vi "XL320_Read Address.vi"(0 "VISA resource name":refnum<visa-resource-name>, 5 "Motor ID (0)":u8, 7 "Address number (0)":u16 max=49, 9 "Number of Addresses to read (1)":u16=1, 11 "Error in (no error)":errorcluster) -> (4 "VISA resource name Out":refnum<visa-resource-name>, 6 "Data Read":u8[](array[numeric]), 10 "Motor Error Status":T1, 15 "error out":errorcluster)   [LabVIEW 2017, in "Dynamixel XL320.lvlib"]
doc: "Reads an arbitrary number of consecutive addresses from a motor's register. This is a Low-Level VI that is used by other VIs."
uses:
  <instrlib>/Dynamixel XL320 (Drivers instrument)/Dynamixel XL320.lvlib
  <instrlib>/Dynamixel XL320 (Drivers instrument)/Public/Motor Operation/Low Level/XL320_Alarm Setting.ctl
  <instrlib>/Dynamixel XL320 (Drivers instrument)/Public/Configure/XL320_Select_Action.ctl
panel:
  # "Ghislain REMY, IUT de Cachan, 2015 December 2015"
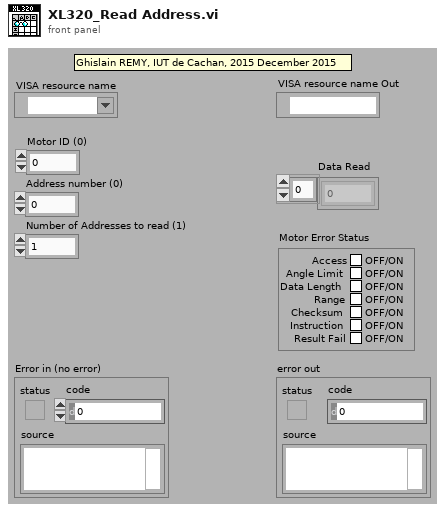
[diagram p1: front panel]
types:
  T1 = typedef "Dynamixel XL320.lvlib/XL320_Alarm Setting.ctl" = cluster{"Access":bool, "Angle Limit":bool, "Data Length":bool, "Range":bool, "Checksum":bool, "Instruction":bool, "Result Fail":bool}
  T2 = cluster{"Boolean array[0]":bool, "Boolean array[1]":bool, "Boolean array[2]":bool, "Boolean array[3]":bool, "Boolean array[4]":bool, "Boolean array[5]":bool, "Boolean array[6]":bool}
  T3 = typedef "Dynamixel XL320.lvlib/XL320_Select_Action.ctl" = u8
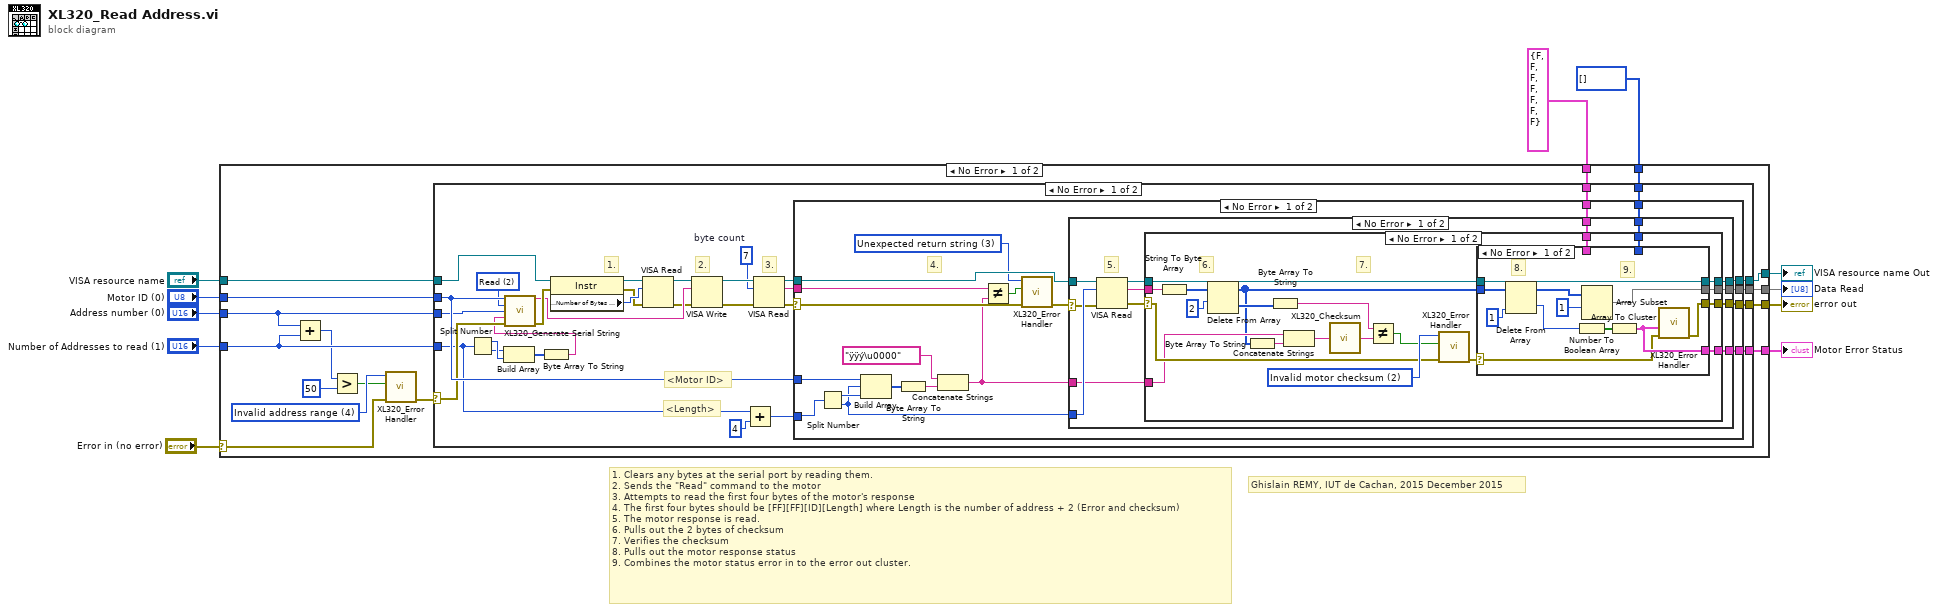
[diagram p0: block diagram]
diagram:
  # "Ghislain REMY, IUT de Cachan, 2015 December 2015"
  # "1. Clears any bytes at the serial port by reading them.\n2. Sends the \"Read\" command to the motor\n3. Attempts to read the first four bytes of the motor's response\n4. The first four bytes should be [FF][FF][ID][Length] where Length is the number of address + 2 (Error and checksum)\n5. The motor response is read.\n6. Pulls out the 2 bytes of checksum\n7. Verifies the checksum\n8. Pulls out the motor response status\n9. Combines the motor status error in to the error out cluster."
  n1 = case shown="No Error" "Error in (no error)" {
    selector: "Error in (no error)" -> [w13 w147]
    tunnel: "Address number (0)" -> [w20 _]
    tunnel: [w23 w145] -> w10
    tunnel: "VISA resource name" -> [w27 w146]
    tunnel: "Number of Addresses to read (1)" -> [w21 _]
    tunnel: "Motor ID (0)" -> [w25 _]
    tunnel: [w26 w146] -> w6
    tunnel: [w24 w147] -> w5
    tunnel: [w22 w144] -> w1
    tunnel: u8[] [] ("unsigned byte array") -> [w17 w145]
    tunnel: T2 {"Boolean array[0]"=FALSE, "Boolean array[1]"=FALSE, "Boolean array[2]"=FALSE, "Boolean array[3]"=FALSE, "Boolean array[4]"=FALSE, "Boolean array[5]"=FALSE, "Boolean array[6]"=FALSE} ("Boolean array") -> [w16 w144]
    frame No Error {
      w15 = u16 4 items=["Scan timeout"=1, "Invalid motor checksum"=2, "Unexpected return string"=3, "Invalid address range"=4] ("Error type")
      n2 = Add(x=w20, y=w21) -> (x+y=w19:u16)
      n3 = Greater?(x=w19, y=u16 50) -> (0:w14:bool)
      n4 = call <instrlib>:"XL320_Error Handler.vi"("error in (no error)"=w13, "Error? (no error)"=w14, "Error type"=w15) -> ("error out"=w12:errorcluster)  [unwired: 8 in]
      n5 = case shown="No Error" w12 {
        selector: w12 -> [w43 w142]
        tunnel: w27 -> [w57 w143]
        tunnel: [w56 w143] -> w26
        tunnel: w25 -> [w45 _]
        tunnel: [w53 w142] -> w24
        tunnel: [w52 w141] -> w23
        tunnel: [w51 w140] -> w22
        tunnel: w21 -> [w34 _]
        tunnel: w20 -> [w44 _]
        tunnel: w17 -> [w47 w141]
        tunnel: w16 -> [w46 w140]
        frame No Error {
          w28 = T3 2 items=["Ping"=1, "Read"=2, "Write"=3, "Registered Write"=4, "Action"=5, "Reset"=6, "Reboot"=8, "Status"=85, "Sync Read"=130, "Sync Write"=131, "Bulk Read"=146, "Bulk Write"=147] ("Select Action")
          w29 = u32 7  # byte count
          # "<Length>"
          # "<Motor ID>"
          # "3."
          # "2."
          # "1."
          n6 = Split Number(x=w34) -> (hi(x)=w36:u8, lo(x)=w35:u8)
          n7 = Build Array(w35, w36) -> (w33:u8[])
          n8 = Byte Array To String(unsigned byte array=w33) -> (string=w32:string)
          n9 = call <instrlib>:"XL320_Generate Serial String.vi"("Motor ID"=w45, "Select Action"=w28, "Address"=w44, "Parameters"=w32, "Error in (no error)"=w43) -> ("Command to Serial"=w41:string, "error out"=w42:errorcluster)  [unwired: 9 in]
          n10 = property class="Instr"(reference=w57, error in=w42) -> (reference out=w54:refnum<visa-resource-name>, error out=w40:errorcluster, "Serial Settings:Number of Bytes at Serial Port"=w55:u32)
          n11 = VISA Read(VISA resource name=w54, byte count=w55, error in (no error)=w40) -> (VISA resource name out=w58:refnum<visa-resource-name>, error out=w39:errorcluster)  [unwired: 2 out]
          n12 = VISA Write(VISA resource name=w58, write buffer=w41, error in (no error)=w39) -> (VISA resource name out=w31:refnum<visa-resource-name>, error out=w30:errorcluster)  [unwired: 1 out]
          n13 = Add(x=w34, y=u16 4) -> (x+y=w37:u16)
          n14 = VISA Read(VISA resource name=w31, byte count=w29, error in (no error)=w30) -> (VISA resource name out=w48:refnum<visa-resource-name>, read buffer=w50:string, error out=w49:errorcluster)  [unwired: 1 out]
          n15 = case shown="No Error" w49 {
            selector: w49 -> [w69 w139]
            tunnel: w37 -> [w63 _]
            tunnel: w45 -> [w67 _]
            tunnel: w50 -> [w61 _]
            tunnel: [w76 w139] -> w53
            tunnel: w48 -> [w78 w138]
            tunnel: [w77 w138] -> w56
            tunnel: [w75 w137] -> w52
            tunnel: [w74 w136] -> w51
            tunnel: w47 -> [w73 w137]
            tunnel: w46 -> [w72 w136]
            frame No Error {
              w71 = u16 3 items=["Scan timeout"=1, "Invalid motor checksum"=2, "Unexpected return string"=3, "Invalid address range"=4] ("Error type")
              # "4."
              n16 = Split Number(x=w63) -> (hi(x)=w64:u8, lo(x)=w59:u8)
              n17 = Build Array(w67, w59, w64) -> (w66:u8[])
              n18 = Byte Array To String(unsigned byte array=w66) -> (string=w65:string)
              n19 = Concatenate Strings("ÿÿý\u0000" ("string"), w65) -> (w60:string)
              n20 = Not Equal?(x=w61, y=w60) -> (x != y?=w70:bool)
              n21 = call <instrlib>:"XL320_Error Handler.vi"("error in (no error)"=w69, "Error? (no error)"=w70, "Error type"=w71) -> ("error out"=w68:errorcluster)  [unwired: 8 in]
              n22 = case shown="No Error" w68 {
                selector: w68 -> [w81 w134]
                tunnel: w78 -> [w91 w135]
                tunnel: [w83 w135] -> w77
                tunnel: [w87 w134] -> w76
                tunnel: w59 -> [w90 _]
                tunnel: w60 -> [w86 _]
                tunnel: [w85 w133] -> w75
                tunnel: [w84 w132] -> w74
                tunnel: w73 -> [w80 w133]
                tunnel: w72 -> [w79 w132]
                frame No Error {
                  # "5."
                  n23 = VISA Read(VISA resource name=w91, byte count=w90, error in (no error)=w81) -> (VISA resource name out=w82:refnum<visa-resource-name>, read buffer=w89:string, error out=w88:errorcluster)  [unwired: 1 out]
                  n24 = case shown="No Error" w88 {
                    selector: w88 -> [w102 w131]
                    tunnel: w89 -> [w110 _]
                    tunnel: [w112 w131] -> w87
                    tunnel: w86 -> [w95 _]
                    tunnel: [w111 w129] -> w85
                    tunnel: [w107 w128] -> w84
                    tunnel: [w109 w130] -> w83
                    tunnel: w82 -> [w108 w130]
                    tunnel: w80 -> [w106 w129]
                    tunnel: w79 -> [w105 w128]
                    frame No Error {
                      w104 = u16 2 items=["Scan timeout"=1, "Invalid motor checksum"=2, "Unexpected return string"=3, "Invalid address range"=4] ("Error type")
                      # "7."
                      # "6."
                      n25 = String To Byte Array(string=w110) -> (unsigned byte array=w93:u8[])
                      n26 = Delete From Array(array=w93, length=2) -> (deleted portion=w100:u8[], array with subset deleted=w92:u8[])  [unwired: 1 in]
                      n27 = Byte Array To String(unsigned byte array=w92) -> (string=w94:string)
                      n28 = Byte Array To String(unsigned byte array=w100) -> (string=w98:string)
                      n29 = Concatenate Strings(w95, w94) -> (w96:string)
                      n30 = call <instrlib>:"XL320_Checksum.vi"("Input String"=w96) -> ("Checksum String"=w97:string)
                      n31 = Not Equal?(x=w98, y=w97) -> (x != y?=w103:bool)
                      n32 = call <instrlib>:"XL320_Error Handler.vi"("error in (no error)"=w102, "Error? (no error)"=w103, "Error type"=w104) -> ("error out"=w101:errorcluster)  [unwired: 8 in]
                      n33 = case shown="No Error" w101 {
                        selector: w101 -> [w118 w126]
                        tunnel: [w113 w125] -> w111
                        tunnel: w92 -> [w122 _]
                        tunnel: [w117 w126] -> w112
                        tunnel: [w123 w127] -> w109
                        tunnel: w108 -> [w123 w127]
                        tunnel: [w119 w124] -> w107
                        tunnel: w106 -> [_ w125]
                        tunnel: w105 -> [_ w124]
                        frame No Error {
                          # "8."
                          # "9."
                          n34 = Delete From Array(array=w122, index=1) -> (deleted portion=w115:u8, array with subset deleted=w114:u8[])  [unwired: 1 in]
                          n35 = Number To Boolean Array(number=w115) -> (Boolean array=w120:bool[])
                          n36 = Array Subset(array=w114, index=1 ("length")) -> (w113:u8[])  [unwired: 1 in]
                          n37 = Array To Cluster(array=w120) -> (cluster=w119:T2)
                          n38 = call <instrlib>:"XL320_Error Handler.vi"("error in (no error)"=w118, "Motor Error Status (none)"=w119) -> ("error out"=w117:errorcluster)  [unwired: 9 in]
                        }
                        frame Error {
                        }
                      }
                    }
                    frame Error {
                    }
                  }
                }
                frame Error {
                }
              }
            }
            frame Error {
            }
          }
        }
        frame Error {
        }
      }
    }
    frame Error {
    }
  }
  "Data Read" <- w10
  "VISA resource name Out" <- w6
  "error out" <- w5
  "Motor Error Status" <- w1
